vi "CustomView.vi"(8 "error in":errorcluster, 10 "view name":string, 11 "repository in":refnum<class "NISE_CEF_Repository.lvclass">) -> (0 "error out":errorcluster, 3 "repository out":refnum<class "NISE_CEF_Repository.lvclass">)   [LabVIEW 2013, in "NISE_CEF_Repository.lvclass"]
doc: "Calls the custom view specified in the view name string. The purpose of this method is to allow adding a Configurator editor without modifying the main VI"
uses:
  NISE_CEF_Repository.lvclass
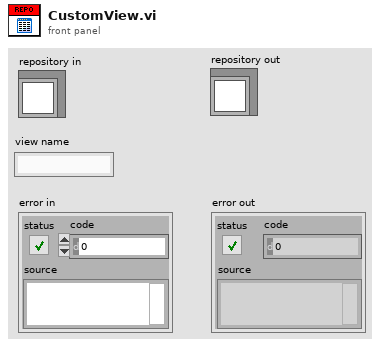
[diagram p1: front panel]
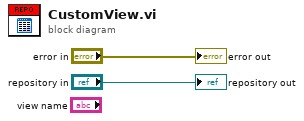
[diagram p0: block diagram]
diagram:
  "repository out" <- "repository in"
  "error out" <- "error in"
